vi "Copy and Update Rev # on APU Setup File.vi"(8 "error in (no error)":errorcluster, 11 "Latest Path in":path) -> (0 "error out":errorcluster, 3 "New Rev Path out":path)   [LabVIEW 2018, in "File IO.lvlib"]
doc: "Finds the latest APU setup file. Copies the file with a new date and/or rev #"
uses:
  File IO.lvlib
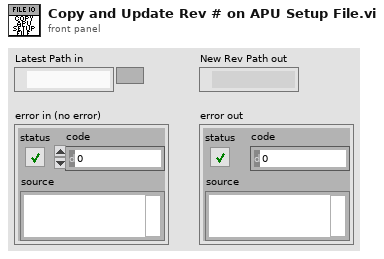
[diagram p1: front panel]
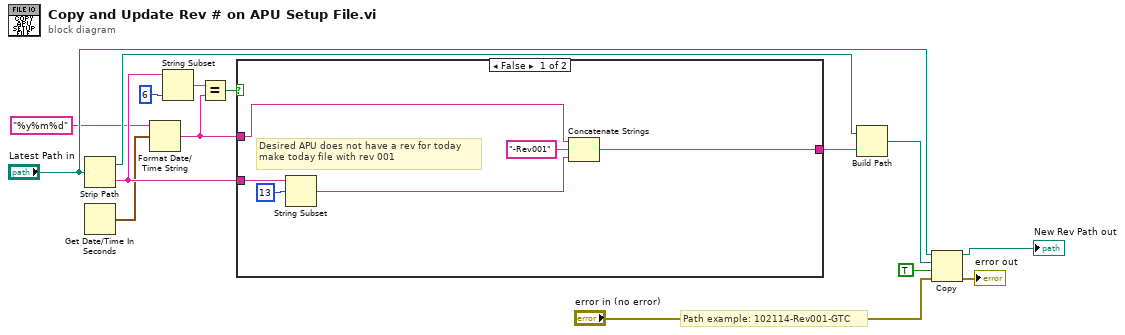
[diagram p0: block diagram]
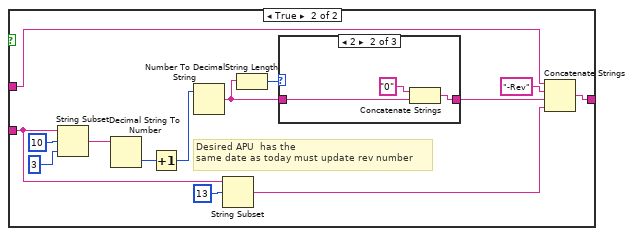
[diagram p2: hidden frame]
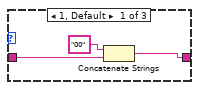
[diagram p3: hidden frame]
diagram:
  # "Path example: 102114-Rev001-GTC"
  n1 = Strip Path(path="Latest Path in") -> (stripped path=w13:path, name=w14:string)
  n2 = Get Date/Time In Seconds() -> (seconds since 1Jan1904=w3:timestamp)
  n3 = Format Date/Time String(time format string (%c)="%y%m%d", seconds (now)=w3) -> (date/time string=w6:string)  [unwired: 1 in]
  n4 = String Subset(string=w14, length (rest)=6 ("length (rest)")) -> (substring=w5:string)  [unwired: 1 in]
  n5 = Equal?(x=w5, y=w6) -> (x = y?=w7:bool)
  n6 = case shown="False" w7 {
    tunnel: w14 -> [w21 w25]
    tunnel: w6 -> [w19 w28]
    tunnel: [w16 w22] -> w9
    frame False {
      # "Desired APU does not have a rev for today\nmake today file with rev 001"
      n7 = String Subset(string=w21, offset (0)=13) -> (substring=w17:string)  [unwired: 1 in]
      n8 = Concatenate Strings(w19, "-Rev001" ("string"), w17) -> (w16:string)
    }
    frame True {
      # "Desired APU  has the \nsame date as today must update rev number"
      n9 = String Subset(string=w25, offset (0)=10, length (rest)=3 ("length (rest)")) -> (substring=w33:string)
      n10 = Decimal String To Number(string=w33) -> (number=w32:i32)  [unwired: 2 in, 1 out]
      n11 = Increment(x=w32) -> (x+1=w31:i32)
      n12 = Number To Decimal String(number=w31) -> (decimal integer string=w29:string)  [unwired: 1 in]
      n13 = String Subset(string=w25, offset (0)=13) -> (substring=w23:string)  [unwired: 1 in]
      n14 = String Length(string=w29) -> (length=w30:i32)
      n15 = case shown="2" w30 {
        tunnel: w29 -> [w38 w41 w42]
        tunnel: [w36 w39 w42] -> w26
        frame 1, Default {
          n16 = Concatenate Strings("00" ("string"), w38) -> (w36:string)
        }
        frame 2 {
          n17 = Concatenate Strings("0" ("string"), w41) -> (w39:string)
        }
        frame 3 {
        }
      }
      n18 = Concatenate Strings(w28, "-Rev" ("string"), w26, w23) -> (w22:string)
    }
  }
  n19 = Build Path(base path=w13, name or relative path=w9) -> (appended path=w10:path)
  n20 = Copy(8:"error in (no error)", 9:TRUE ("overwrite (F)"), 10:w10, 11:"Latest Path in") -> (0:→"error out":errorcluster, 3:→"New Rev Path out":path)  [unwired: 1 in, 1 out]
